vi "Tx Streaming (Host).vi"() -> ()   [LabVIEW 2021]
doc: "This template is for the Simple NI-USRP Streaming design, a design that shows the basics of streaming data to and from an NI USRP-294x/295x device. Refer to the block diagram for more information about how to use this template."
uses:
  <vilib>/userDefined/Silver/nirio_resource_slv.ctl
  SubVIs/Start Trigger.ctl
  <vilib>/Utility/error.llb/DialogType.ctl
panel:
  in  "config tab":enum32{"Tx Configuration"}(tab)
  in  "tx config":T2={"rf enable 0"=TRUE, "rf config 0"={"antenna"="TX1", "frequency"=2000000000.0, "lo frequency"=-1.0, "level"=0.0}, "rf enable 1"=TRUE, "rf config 1"={"antenna"="TX1", "frequency"=2000000000.0, "lo frequency"=-1.0, "level"=0.0}, "transfer mode"=enum."Finite", "sample rate"=10000000.0, "number of samples"=8192, "start trigger"=enum."Immediate", "tone frequency"=100000.0} {"tone frequency" format="%#.3pHz"; "sample rate" format="%#.3pS/s"; "rf config 0"."level" format="%#_gdBm"; "rf config 0"."lo frequency" format="%#.3pHz"; "rf config 0"."frequency" format="%#.3pHz"; "rf config 1"."level" format="%#_gdBm"; "rf config 1"."lo frequency" format="%#.3pHz"; "rf config 1"."frequency" format="%#.3pHz"}
  in  "tx.stop":bool
  out "generating":bool caption="Generating"
  in  "USRP RIO device":T3="RIO0" caption="USRP RIO Device"
  in  "reference frequency source":string(combo)="Internal" caption="Reference Frequency Source"
  in  "indicator tab":T4(tab)
  out "tx.output waveform":waveform(dbl)[](graph) caption="Output Waveform"
  out "tx.coerced config":T5 caption="Tx" {"coerced sample rates" format="%#.3pS/s"; "coerced levels" format="%#.3gdBm"; "coerced lo frequencies" format="%#.3pHz"; "coerced frequencies" format="%#.3pHz"}
  # "This template is for the Simple NI-USRP Streaming design, a design that shows the basics of streaming data on a USRP RIO device. See the block diagram for more information on how to use this template."
  # "Simple Tx Streaming"
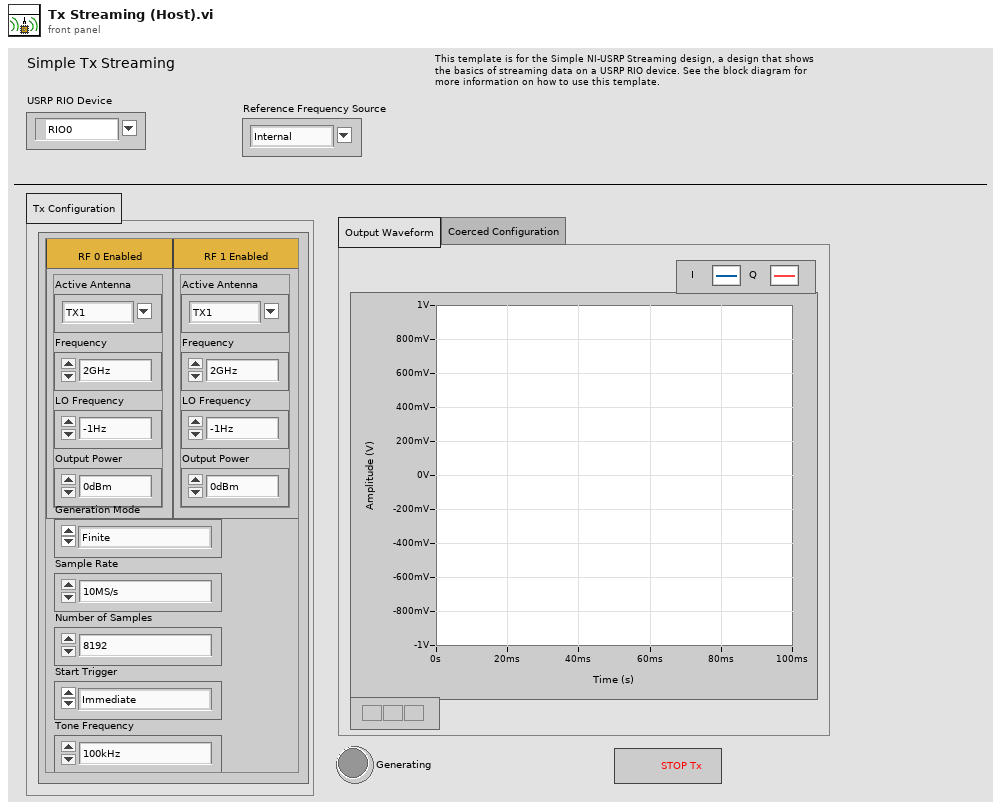
[diagram p1: front panel]
types:
  T1 = typedef "Start Trigger.ctl" = enum8{"Software", "Digital Edge", "Rx Start Trigger", "Tx Start Trigger", "Immediate", "Future Time Event"}
  T2 = cluster{"rf enable 0":bool, "rf config 0":cluster{"antenna":string, "frequency":dbl, "lo frequency":dbl, "level":dbl}, "rf enable 1":bool, "rf config 1":cluster{"antenna":string, "frequency":dbl, "lo frequency":dbl, "level":dbl}, "transfer mode":enum16{"Finite", "Continuous"}, "sample rate":dbl, "number of samples":u32, "start trigger":T1, "tone frequency":dbl}
  T3 = typedef "nirio_resource_slv.ctl" = tag
  T4 = enum32{"Output Waveform", "Coerced Configuration"}
  T5 = cluster{"coerced frequencies":dbl[], "coerced lo frequencies":dbl[], "coerced levels":dbl[], "coerced sample rates":dbl[]}
  T6 = typedef "DialogType.ctl" = u16
  T7 = typedef "Tx Channels.ctl" = cluster{"tx config":cluster{"channel configuration":cluster{"channel enable":bool, "channel configuration":cluster{"antenna":string, "frequency":dbl, "lo frequency":dbl, "level":dbl}}[], "transfer mode":enum16{"Finite", "Continuous"}, "sample rate":dbl, "number of samples":u32, "start trigger":T1, "tone frequency":dbl}, "reference frequency source":string, "tx.data source":enum16{"SFP Port 0", "SFP Port 1", "Host"}, "tx.enabled channels":string[], "I":i16[], "Q":i16[], "tx.coerced configurations":cluster{"coerced frequencies":dbl[], "coerced lo frequencies":dbl[], "coerced levels":dbl[], "coerced sample rates":dbl[]}}
  T8 = typedef "niUsrpRio Config v1 Host.lvlib/niUsrpRio Session.ctl" = cluster{"FPGA Interface":refnum<k20>, "RIO Interface Number":u32, "Data Clock Rate":u32, "FPGA Data Clock Rate":u32, "Global Settings Register Bus":T9, "Radio 0 Settings Register Bus":T9, "Radio 1 Settings Register Bus":T9, "Radio Settings Bus Semaphore":T10, "DB Queues":T11[], "Characterization Data Valid?":bool, "EEPROM Header":T12, "Device Data Header":T13, "EEPROM Characterization Header":T14, "Characterization Data":T15[], "FPGA Current Version":u32, "FPGA Oldest Compatible Version":u32, "Fixed Logic Current Version":u32, "Fixed Logic Oldest Compatible Version":u32, "FPGA Radio Settings Bus Current Version":u32, "FPGA Radio Settings Bus Oldest Compatible Version":u32, "FPGA Board Config Current Version":u32, "FPGA Board Config Oldest Compatible Version":u32, "Daughterboard Clock Rate":u32, "daughterboard configuration session handles":u64[]}
  T9 = typedef "niInstr Register Bus v0 Host.lvlib/Register Bus Session.ctl" = refnum<queue>
  T10 = typedef "Semaphore RefNum" = refnum<k1>
  T11 = typedef "niUsrpRio Config v1 Host.lvlib/DB Queue Reference.ctl" = refnum<queue>
  T12 = typedef "niUsrpRio Config v1 Host.lvlib/EEPROM Header.ctl" = cluster{"Checksum":u32, "Product Code":u16, "Hardware Current Version":u16, "Hardware Oldest Compatible Version":u16, "EEPROM Map Current Version":u16, "EEPROM Map Oldest Compatible Version":u16, "User Password":string, "Pointer to Factory Header":u32, "Pointer to User Header":u32, "Recommended Interval":u16, "Number of Reserved Bytes":i32, "Number of Daughterboards":u8, "Daughterboard IDs":u16[], "Daughterboard Serial Numbers":string[]}
  T13 = typedef "niUsrpRio Config v1 Host.lvlib/EEPROM Device Data Header.ctl" = cluster{"Checksum":u32, "Number of Channels":u8, "Number of Gain Settings":u16[], "Pointer to Characterization Data":u32[], "Number of Reserved Bytes":i32, "Number of Frequencies":u16[]}
  T14 = typedef "niUsrpRio Config v1 Host.lvlib/EEPROM Characterization Header.ctl" = cluster{"Checksum":u32, "Date":timestamp, "Temperature":sgl, "Misc. Info":string, "Pointer to Device Data Header":u32, "Number of Reserved Bytes":i32}
  T15 = typedef "niUsrpRio Config v1 Host.lvlib/Characterization Data.ctl" = cluster{"Gains[dB]":dbl[], "Frequencies [Hz]":dbl[], "IQ Imbalance Table":T16[], "Measured Gains[dB]":dbl[][]}
  T16 = typedef "niUsrpRio Config v1 Host.lvlib/IQ Imbalance.ctl" = cluster{"Gain Imbalance [linear]":dbl, "Phase Imbalance [radians]":dbl, "Offset":cdb}
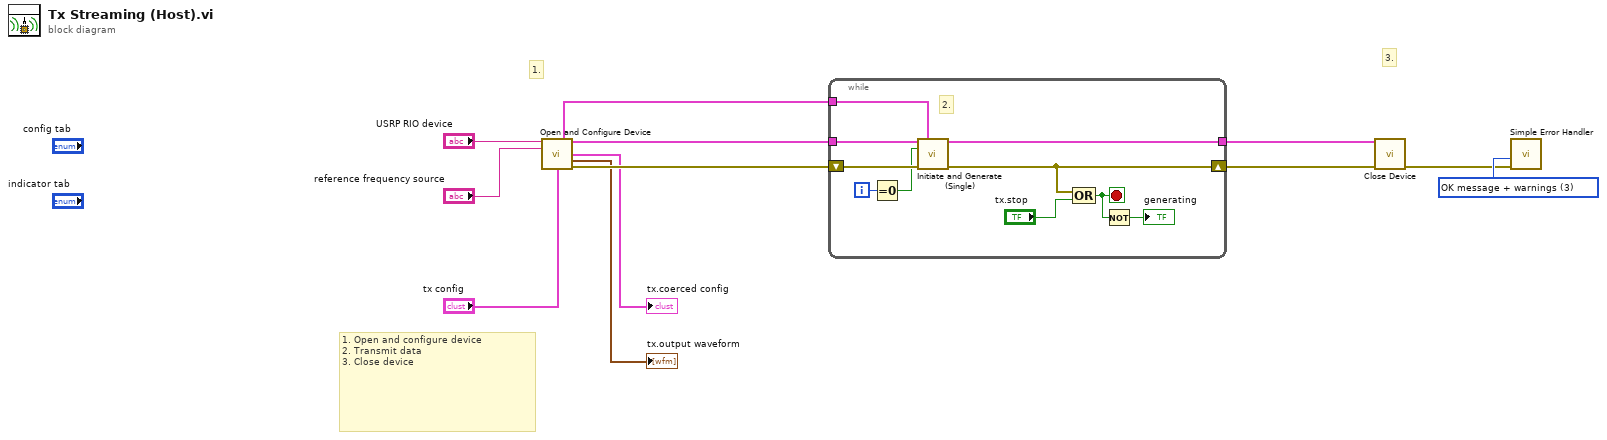
[diagram p0: block diagram]
diagram:
  w11 = T6 3 items=["no dialog", "OK message", "continue or stop message", "OK message + warnings", "continue/stop + warnings"] ("type of dialog (OK msg:1)")
  # "3."
  # "1. Open and configure device\n2. Transmit data\n3. Close device"
  # "1."
  n1 = call "Open and Configure Device.vi"("USRP RIO Device"="USRP RIO device", "reference frequency source"="reference frequency source", "tx config"="tx config") -> ("tx channels"=w6:T7, "niUsrpRio Session (out)"=w2:T8, "tx.coerced configurations"=→"tx.coerced config":T5, "tx.output waveform"=→"tx.output waveform":waveform(dbl)[], "error out"=w12:errorcluster)  [unwired: 6 in, 2 out]
  n2 = while {
    tunnel: w2 -> [w20]
    tunnel: w6 -> [w15]
    tunnel: [w14] -> w1
    shift-right: [w18] -> w4
    shift-left: w12 -> [w19]
    i -> [w17]
    stop <- w16 stop-if-true
    # "2."
    # "Acquire and Fetch a waveform"
    n3 = Equal To 0?(x=w17) -> (x = 0?=w13:bool)
    n4 = call "Initiate and Generate (Single).vi"("niUsrpRio Session"=w20, "tx channels"=w15, "first iteration"=w13, "error in"=w19) -> ("niUsrpRio Session (out)"=w14:T8, "error out"=w18:errorcluster)  [unwired: 10 in]
    n5 = Compound Arithmetic op=OR(w18, "tx.stop") -> (w16:bool)
    n6 = Not(x=w16) -> (.not. x?=→"generating":bool)
  }
  n7 = call "Close Device.vi"("niUsrpRio Session"=w1, "error in"=w4) -> ("error out"=w10:errorcluster)  [unwired: 13 in]
  n8 = call <vilib>:"Simple Error Handler.vi"("type of dialog (OK msg:1)"=w11, "error in (no error)"=w10) -> ()  [unwired: 3 in, 5 out]
